vi "myRIO_BRig_RT_dataExp_TPB_min__L.vi"() -> (2 "output_TPB_min__L":i32)   [LabVIEW 2014]
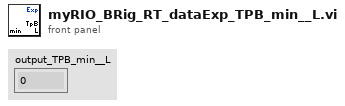
[diagram p1: front panel]
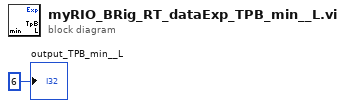
[diagram p0: block diagram]
diagram:
  "output_TPB_min__L" <- 6 ("output_iBlock")
